vi "照抄版'heart.vi"() -> ()   [LabVIEW 2013]
uses:
  <vilib>/measure/mamon.llb/Waveform Peak Detection for N Chan.vi
  <vilib>/measure/NI_MAPro.lvlib
panel:
  out "Waveform Graph":dynamicdata(graph)
  out "Waveform Chart":dynamicdata(graph)
  in  "stop":bool
  out "heart rate":dbl
  out "frequence":dbl
  out "Scalar":dbl
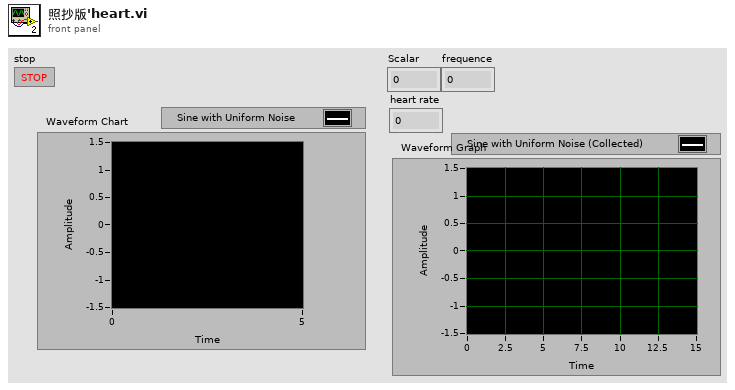
[diagram p1: front panel]
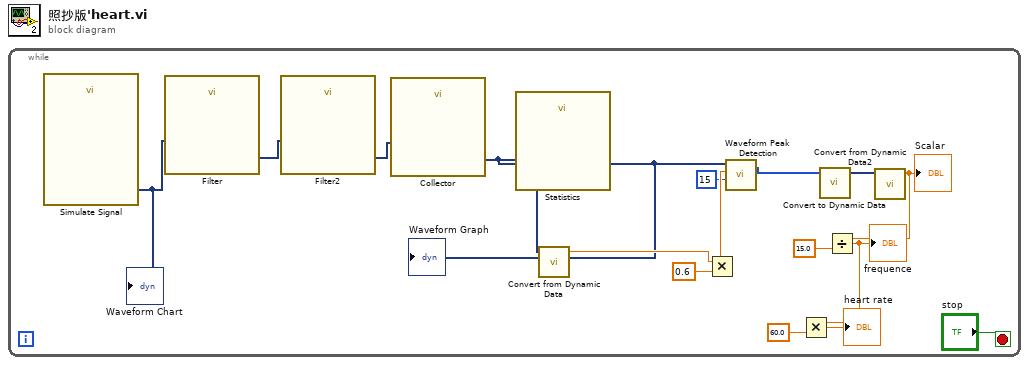
[diagram p0: block diagram]
diagram:
  n1 = while {
    stop <- "stop" stop-if-true
    n2 = call "Simulate Signal"() -> ("Sine with Uniform Noise"=w4:dynamicdata)  [unwired: 14 in, 1 out]
    "Waveform Chart" <- w4
    n3 = call "Filter"("Signal"=w4) -> ("Filtered Signal"=w17:dynamicdata)  [unwired: 9 in, 1 out]
    n4 = call "Filter2"("Signal"=w17) -> ("Filtered Signal"=w16:dynamicdata)  [unwired: 9 in, 1 out]
    n5 = call "Collector"("Signals"=w16) -> ("Collected Signals"=w1:dynamicdata)  [unwired: 9 in, 1 out]
    "Waveform Graph" <- w1
    n6 = call "Statistics"("Signals"=w1) -> ("Maximum"=w2:dynamicdata)  [unwired: 25 in, 1 out]
    n7 = call "Convert from Dynamic Data"("Dynamic Data Type"=w2) -> ("Scalar"=w14:dbl)  [unwired: 3 in]
    n8 = Multiply(x=w14, y=0.6) -> (x*y=w13:dbl)
    n9 = call-poly <vilib>:"Waveform Peak Detection.vi"("width"=15, "threshold"=w13, "Signals In"=w1) -> ("# found"=w10:i32[])  [unwired: 4 in, 4 out]
    n10 = call "Convert to Dynamic Data"("Array"=w10) -> ("Dynamic Data Type"=w11:dynamicdata)  [unwired: 3 in]
    n11 = call "Convert from Dynamic Data2"("Dynamic Data Type"=w11) -> ("Scalar"=w8:dbl)  [unwired: 3 in]
    "Scalar" <- w8
    n12 = Divide(x=w8, y=15.0) -> (x/y=w3:dbl)
    "frequence" <- w3
    n13 = Multiply(x=w3, y=60.0) -> (x*y=→"heart rate":dbl)
  }
